vi "main - Server.vi"() -> ()   [LabVIEW 2024]
uses:
  <vilib>/Instr/_visa.llb/VISA Configure Serial Port (Instr).vi
panel:
  in  "Clr?":bool
  out "Iterations":i32=291
  in  "Tx":bool
  in  "Tx String":string
  in  "Serial Port":refnum<visa-resource-name>="COM6"
  in  "Clear":bool
  out "error out":errorcluster={"status"=FALSE, "code"=1073676294, "source"="VISA Read in main - Server.vi"}
  in  "Stop":bool
  out "Console":string="ets Jul 29 2019 12:21:46\r\n\r\nrst:0x1 (POWERON_RESET),boot:0x1e (SPI_FAST_FLASH_BOOT)\r\nconfigsip: 0, SPIWP:0xee\r\nclk_drv:0x00,q_drv:0x00,d_drv:0x00,cs0_drv:0x00,hd_drv:0x00,wp_drv:0x00\r\nmode:DIO, clock div:2\r\nload:0x3fff0030,len:6276\r\nload:0x40078000,len:15716\r\nload:0x40080400,len:4\r\nho 8 tail 4 room 4\r\nload:0x40080404,len:3860\r\nentry 0x4008063c\r\nI (31) boot: ESP-IDF v5.4-dirty 2nd stage bootloader\r\nI (31) boot: compile time Mar  8 2025 15:10:28\r\nI (31) boot: Multicore bootloader\r\nI (33) boot: chip revision: v3.1\r\nI (36) boot.esp32: SPI Speed      : 40MHz\r\nI (39) boot.esp32: SPI Mode       : DIO\r\nI (43) boot.esp32: SPI Flash Size : 2MB\r\nI (47) boot: Enabling RNG early entropy source...\r\nI (51) boot: Partition Table:\r\nI (54) boot: ## Label            Usage          Type ST Offset   Length\r\nI (60) boot:  0 nvs              WiFi data        01 02 00009000 00006000\r\nI (66) boot:  1 phy_init         RF data          01 01 0000f000 00001000\r\nI (73) boot:  2 factory          factory app      00 00 00010000 00100000\r\nI (80) boot: End of partition table\r\nI (83) esp_image: segment 0: paddr=00010020 vaddr=3f400020 size=1fa84h (129668) map\r\nI (135) esp_image: segment 1: paddr=0002faac vaddr=3ff80000 size=0001ch (    28) load\r\nI (135) esp_image: segment 2: paddr=0002fad0 vaddr=3ffbdb60 size=00548h (  1352) load\r\nI (139) esp_image: segment 3: paddr=00030020 vaddr=400d0020 size=7cc88h (511112) map\r\nI (321) esp_image: segment 4: paddr=000accb0 vaddr=3ffbe0a8 size=04698h ( 18072) load\r\nI (327) esp_image: segment 5: paddr=000b1350 vaddr=40080000 size=187c8h (100296) load\r\nI (378) boot: Loaded app from partition at offset 0x10000\r\nI (379) boot: Disabling RNG early entropy source...\r\nI (389) cpu_start: Multicore app\r\nI (397) cpu_start: Pro cpu start user code\r\nI (397) cpu_start: cpu freq: 160000000 Hz\r\nI (397) app_init: Application information:\r\nI (398) app_init: Project name:     ble_spp_server_demo\r\nI (402) app_init: App version:      r0\r\nI (406) app_init: Compile time:     Mar  8 2025 15:09:51\r\nI (411) app_init: ELF file SHA256:  44aff87ec...\r\nI (415) app_init: ESP-IDF:          v5.4-dirty\r\nI (419) efuse_init: Min chip rev:     v0.0\r\nI (423) efuse_init: Max chip rev:     v3.99 \r\nI (427) efuse_init: Chip rev:         v3.1\r\nI (431) heap_init: Initializing. RAM available for dynamic allocation:\r\nI (438) heap_init: At 3FFAFF10 len 000000F0 (0 KiB): DRAM\r\nI (442) heap_init: At 3FFB6388 len 00001C78 (7 KiB): DRAM\r\nI (448) heap_init: At 3FFB9A20 len 00004108 (16 KiB): DRAM\r\nI (453) heap_init: At 3FFC7218 len 00018DE8 (99 KiB): DRAM\r\nI (458) heap_init: At 3FFE0440 len 00003AE0 (14 KiB): D/IRAM\r\nI (463) heap_init: At 3FFE4350 len 0001BCB0 (111 KiB): D/IRAM\r\nI (469) heap_init: At 400987C8 len 00007838 (30 KiB): IRAM\r\nI (476) spi_flash: detected chip: generic\r\nI (478) spi_flash: flash io: dio\r\nW (481) spi_flash: Detected size(4096k) larger than the size in the binary image header(2048k). Using the size in the binary image header.\r\nI (494) coexist: coex firmware version: 49a8cdc\r\nI (498) main_task: Started on CPU0\r\nI (508) main_task: Calling app_main()\r\nI (518) BTDM_INIT: BT controller compile version [20b459d]\r\nI (518) BTDM_INIT: Bluetooth MAC: 48:e7:29:a3:b6:52\r\nI (518) phy_init: phy_version 4840,02e0d70,Sep  2 2024,19:39:07\r\nI (828) GATTS_SPP_DEMO: app_main init bluetooth\r\nI (908) GATTS_SPP_DEMO: EVT 0, gatts if 3\r\nI (908) GATTS_SPP_DEMO: event = 0\r\nI (908) GATTS_SPP_DEMO: gatts_profile_event_handler 655\r\nI (908) GATTS_SPP_DEMO: gatts_profile_event_handler 658\r\nI (908) GATTS_SPP_DEMO: gatts_profile_event_handler 661\r\nI (918) uart: queue free spaces: 10\r\nI (918) GATTS_SPP_DEMO: EVT 22, gatts if 3\r\nI (928) GATTS_SPP_DEMO: event = 16\r\nI (928) GATTS_SPP_DEMO: The number handle =b\r\nI (928) GATTS_SPP_DEMO: GAP_EVT, event 4\r\nI (938) GATTS_SPI (948) GATTS_SPP_DEMO: GAP_EVT, event 6\r\nI (948) main_task: Returned from app_main()\r\nI (6208) GATTS_SPP_DEMO: EVT 14, gatts if 3\r\nI (6208) GATTS_SPP_DEMO: event = e\r\nI (6258) GATTS_SPP_DEMO: GAP_EVT, event 21\r\nI (7158) GATTS_SPP_DEMO: EVT 4, gatts if 3\r\nI (7158) GATTS_SPP_DEMO: event = 4\r\nI (7308) GATTS_SPP_DEMO: EVT 2, gatts if 3\r\nI (7308) GATTS_SPP_DEMO: event = 2\r\nI (7308) GATTS_SPP_DEMO: gatts_profile_event_handler():\r\n  //----------------------------------------------------------------------------------------------------//\r\nI (7318) GATTS_SPP_DEMO: Write Value: (\u0001)\r\nI (7318) GATTS_SPP_DEMO: ESP_GATTS_WRITE_EVT : handle = 5\r\nI (7408) GATTS_SPP_DEMO: EVT 2, gatts if 3\r\nI (7408) GATTS_SPP_DEMO: event = 2\r\nI (7408) GATTS_SPP_DEMO: gatts_profile_event_handler():\r\n  //----------------------------------------------------------------------------------------------------//\r\nI (7418) GATTS_SPP_DEMO: Write Value: (\u0001)\r\nI (7418) GATTS_SPP_DEMO: ESP_GATTS_WRITE_EVT : handle = 10\r\nI (13748) GATTS_SPP_DEMO: EVT 5, gatts if 3\r\nI (13748) GATTS_SPP_DEMO: event = 5\r\n"
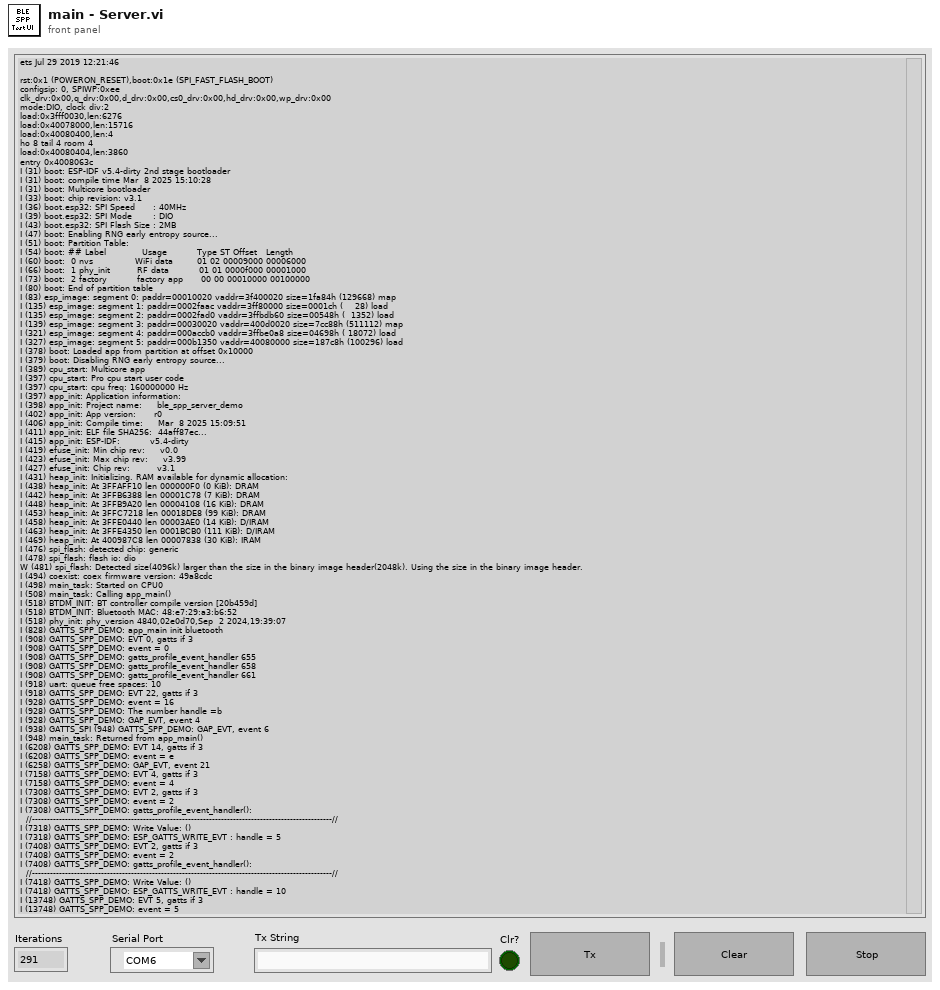
[diagram p1: front panel]
types:
  T1 = enum8{"Enabled", "Disabled", "Disabled and Grayed Out"}
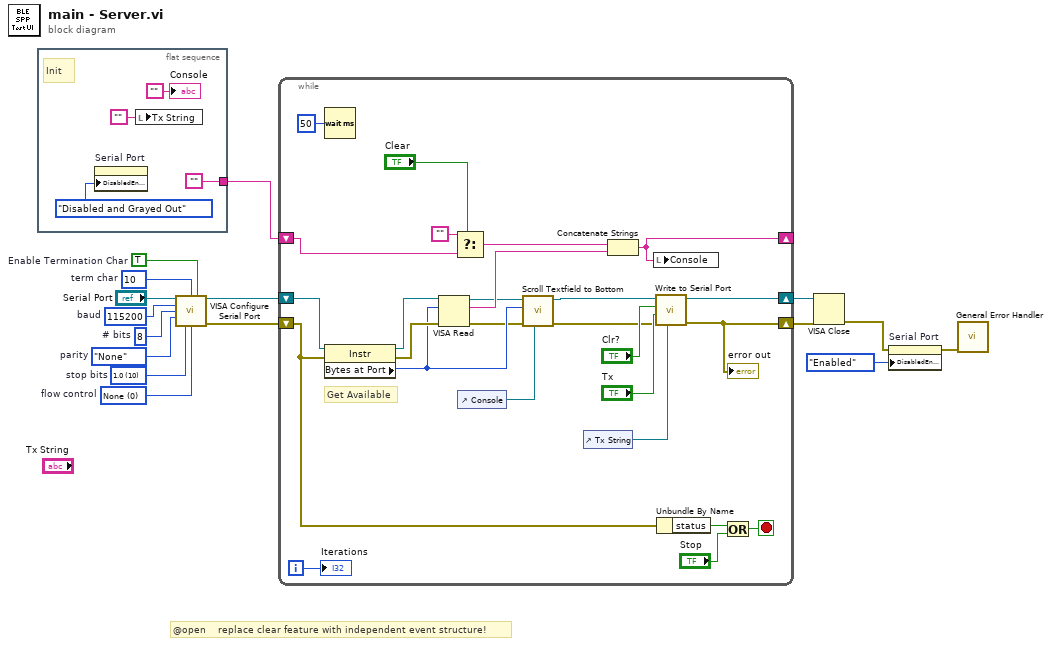
[diagram p0: block diagram]
diagram:
  w10 = u8 10  # term char
  w11 = u16 0 items=["None", "XON/XOFF", "RTS/CTS", "XON/XOFF & RTS/CTS", "DTR/DSR", "XON/XOFF & DTR/DSR"]  # flow control
  w12 = TRUE  # Enable Termination Char
  w13 = u16 10 items=["1.0"=10, "1.5"=15, "2.0"=20]  # stop bits
  w14 = enum16{"None", "Odd", "Even", "Mark", "Space"}."None"  # parity
  w15 = u16 8  # # bits
  w16 = u32 115200  # baud
  # "@open    replace clear feature with independent event structure!"
  n1 = flat-sequence {
    tunnel: [""] -> w4
    frame #0 {
      # "Init"
      n2 = property on="Serial Port" class="VISAName"("DisabledEnum"=T1."Disabled and Grayed Out" ("Disabled")) -> ()  [unwired: 2 in, 2 out]
      n3 = local write "Tx String"("") -> ()
      "Console" <- ""
    }
  }
  n4 = call-poly "VISA Configure Serial Port"("VISA resource name"="Serial Port", "termination char\n(0xA = '\\n' = LF)"=w10, "Enable Termination\nChar (T)"=w12, "baud rate (9600)"=w16, "data bits (8)"=w15, "parity (0:none)"=w14, "stop bits (10: 1 bit)"=w13, "flow control (0:none)"=w11) -> ("VISA resource name out"=w9:refnum<visa-resource-name>, "error out"=w8:errorcluster)  [unwired: 6 in]
  n5 = while {
    shift-right: [w29] -> w6
    shift-left: w9 -> [w38]
    shift-right: [w31] -> w7
    shift-left: w8 -> [w35]
    shift-right: [w39] -> _
    shift-left: w4 -> [w42]
    i -> [w26]
    stop <- w44 stop-if-true
    # "Get Available"
    n6 = Wait (ms)(milliseconds to wait=u32 50) -> ()  [unwired: 1 out]
    n7 = property class="Instr"(reference=w38, error in=w35) -> (reference out=w37:refnum<visa-resource-name>, error out=w36:errorcluster, "Bytes at Port"=w33:u32)
    n8 = VISA Read(VISA resource name=w37, byte count=w33, error in (no error)=w36) -> (VISA resource name out=w22:refnum<visa-resource-name>, read buffer=w41:string, error out=w32:errorcluster)  [unwired: 1 out]
    n9 = Select(t="", s="Clear", f=w42) -> (s? t:f=w40:string)
    n10 = control-ref of="Console"() -> (w28:refnum<vi>)
    n11 = call "Scroll Textfield to Bottom.vi"("Console String"=w28, "error in (no error)"=w32, "Bytes at Serial Port"=w33, "VISA refnum in"=w22) -> ("error out"=w24:errorcluster, "VISA refnum out"=w23:refnum<visa-resource-name>)  [unwired: 6 in]
    n12 = control-ref of="Tx String"() -> (w27:refnum<vi>)
    n13 = Concatenate Strings(w40, w41) -> (w39:string)
    n14 = local write "Console"(w39) -> ()
    n15 = call "Write to Serial Port.vi"("Tx String"=w27, "error in (no error)"=w24, "Transmit?"="Tx", "Clear after send?"="Clr?", "VISA refnum in"=w23) -> ("error out"=w31:errorcluster, "VISA refnum out"=w29:refnum<visa-resource-name>)  [unwired: 5 in]
    "error out" <- w31
    n16 = Unbundle By Name(w35) -> ("status"=w46:bool)
    n17 = Or(x=w46, y="Stop") -> (x .or. y?=w44:bool)
    "Iterations" <- w26
  }
  n18 = VISA Close(VISA resource name=w6, error in (no error)=w7) -> (error out=w2:errorcluster)
  n19 = property on="Serial Port" class="VISAName"(error in=w2, "DisabledEnum"=T1."Enabled" ("Disabled")) -> (error out=w3:errorcluster)  [unwired: 1 in, 1 out]
  n20 = call <vilib>:"General Error Handler.vi"("error in (no error)"=w3) -> ()  [unwired: 10 in, 5 out]
